vi "TestResultSave.vi"(10 "TestResultSummary":T1={"auto get refer point"=FALSE, "width1"=0, "width2"=0, "show_TDD11"=[], "show_TDD22"=[], "test time"=["2016/11/14 11:59:03"], "show_impspec"=[], "TestResult"=[], "FileName"="", "FileVersion"=""}, 11 "FileSavePath":path=path "d:/bb.ini") -> ()   [LabVIEW 2011]
uses:
  <vilib>/Utility/config.llb/NI_LVConfig.lvlib
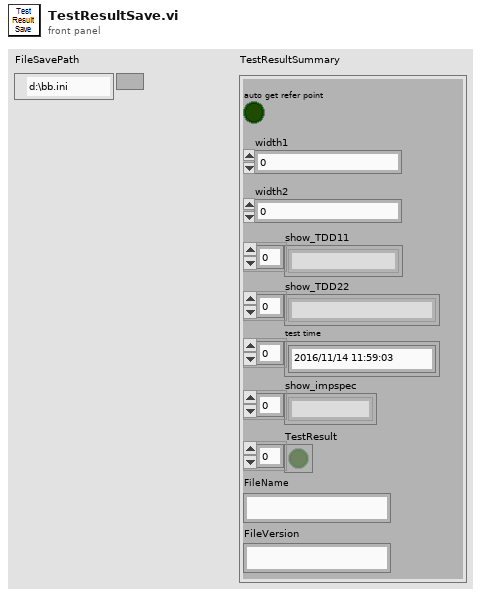
[diagram p1: front panel]
types:
  T1 = cluster{"auto get refer point":bool, "width1":i32, "width2":i32, "show_TDD11":string[], "show_TDD22":string[], "test time":string[], "show_impspec":string[], "TestResult":bool[], "FileName":string, "FileVersion":string}
  T2 = typedef "NI_LVConfig.lvlib/Config Data RefNum.ctl" = refnum<k1>
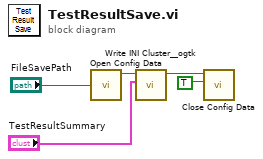
[diagram p0: block diagram]
diagram:
  n1 = call <vilib>:"Open Config Data.vi"("configuration file path"="FileSavePath") -> ("refnum"=w5:T2)  [unwired: 8 in, 2 out]
  n2 = call <userlib>:"Write INI Cluster__ogtk.vi"("INI Fomatted Cluster"="TestResultSummary", "refnum"=w5) -> ("dup refnum"=w3:T2)  [unwired: 8 in, 1 out]
  n3 = call <vilib>:"Close Config Data.vi"("write file if changed (T)"=TRUE, "refnum"=w3) -> ()  [unwired: 8 in, 2 out]
